vi "cRIO Read Serial Number.vi"(8 "error in (no error)":errorcluster, 11 "Refnum in":T1) -> (0 "error out":errorcluster, 2 "Serial Number":string, 3 "Refnum out":T1)   [LabVIEW 2017, in "cRIODetectHW.lvlib"]
uses:
  <vilib>/addons/cRIODetectHW/cRIODetectHW.lvlib
  <vilib>/addons/cRIODetectHW/control/FPGARef.ctl
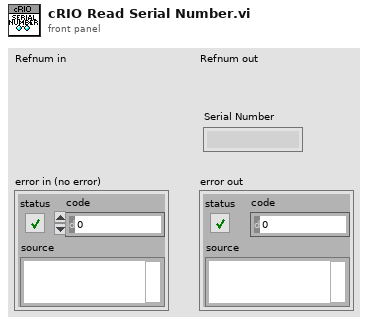
[diagram p1: front panel]
types:
  T1 = typedef "cRIODetectHW.lvlib/FPGARef.ctl" = refnum<k20>
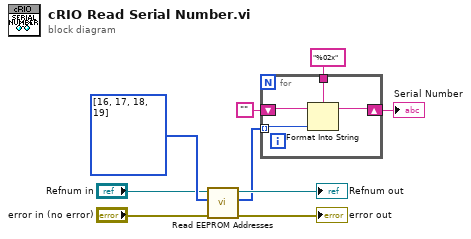
[diagram p0: block diagram]
diagram:
  n1 = call <vilib>:"Read EEPROM Addresses.vi"("error in (no error)"="error in (no error)", "Addresses"=u16[] [16, 17, 18, 19], "Refnum in"="Refnum in") -> ("error out"=→"error out":errorcluster, "Data"=w3:u8[], "Refnum out"=→"Refnum out":T1)  [unwired: 6 in]
  n2 = for {
    tunnel: "%02x" ("format string") -> [w13]
    tunnel: w3 -> [w12] mode=indexing
    shift-right: [w11] -> w1
    shift-left: "" -> [w10]
    n3 = Format Into String(format string=w13, initial string=w10, w12) -> (resulting string=w11:string)  [unwired: 1 in, 1 out]
  }
  "Serial Number" <- w1
